vi "timeval to timestamp.vi"(11 "timeval":T1) -> (3 "timestamp":timestamp)   [LabVIEW 2020, in "libpcaplv.lvlib"]
uses:
  libpcaplv.lvlib
  _typedefs/timeval_type_x64.ctl
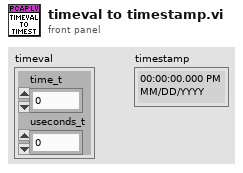
[diagram p1: front panel]
types:
  T1 = typedef "libpcaplv.lvlib/timeval_type_x64.ctl" = cluster{"time_t":u64, "useconds_t":u64}
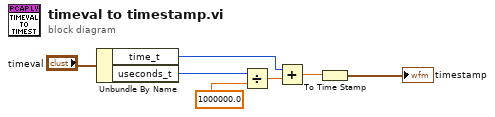
[diagram p0: block diagram]
diagram:
  n1 = Unbundle By Name("timeval") -> ("time_t"=w3:u64, "useconds_t"=w5:u64)
  n2 = Divide(x=w5, y=1000000.0) -> (x/y=w4:dbl)
  n3 = Add(x=w3, y=w4) -> (x+y=w2:dbl)
  n4 = To Time Stamp(1:w2) -> (0:→"timestamp":timestamp)
